vi "AI_InstantAI v2.vi"() -> ()   [LabVIEW 2013]
uses:
  <vilib>/Platform/TimedLoop/XDataNode/timing_clust.ctl
  <vilib>/Platform/TimedLoop/XDataNode/nitl_modes.ctl
  <vilib>/Platform/TimedLoop/XDataNode/wakeup.ctl
  <vilib>/platform/TimedLoop/XDataNode/XDataNode.xnode
  <vilib>/Platform/TimedLoop/XDataNode/XDNodeRunTimeDep.lvlib
panel:
  in  "Samples":i32
  out "loop time":dbl format="%.6g"
  in  "Tab Control":enum32{"Graph0", "Graph1", "Graph2"}(tab)
  out "Graph0":dbl[][](graph)
  out "Ch0":dbl[](array[numeric])
  out "Ch1":dbl[](array[numeric])
  out "Ch2":dbl[](array[numeric])
  out "Ch3":dbl[](array[numeric])
  out "Ch4":dbl[](array[numeric])
  out "Ch5":dbl[](array[numeric])
  out "Ch6":dbl[](array[numeric])
  out "Ch7":dbl[](array[numeric])
  out "error 0":errorcluster
  out "Ch7-1":dbl[](array[numeric])
  out "Ch6-1":dbl[](array[numeric])
  out "Ch5-1":dbl[](array[numeric])
  out "Ch4-1":dbl[](array[numeric])
  out "Ch3-1":dbl[](array[numeric])
  out "Ch2-1":dbl[](array[numeric])
  out "Ch1-1":dbl[](array[numeric])
  out "Ch0-1":dbl[](array[numeric])
  out "error 1":errorcluster
  out "Graph1":dbl[][](graph)
  out "loops":bool
  in  "stop":bool
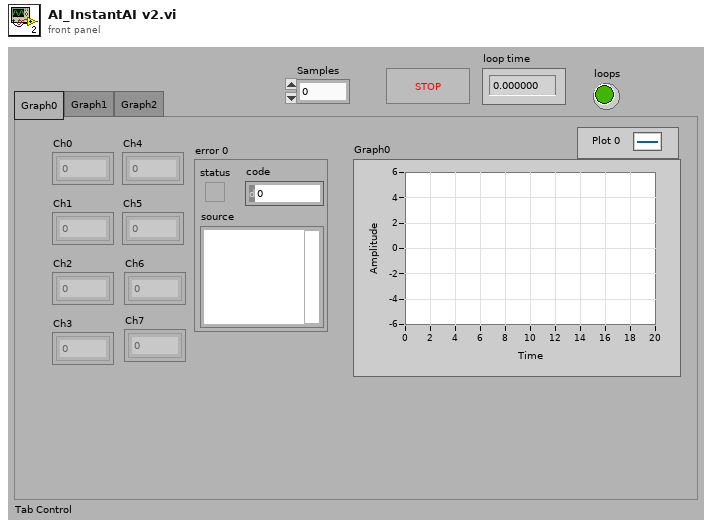
[diagram p1: front panel]
types:
  T1 = typedef "XDNodeRunTimeDep.lvlib/timing_clust.ctl" = cluster{"Expected End [f-1]":u64, "Actual End [f-1]":u64, "Finished Late? [f-1]":bool, "Expected End [i-1]":u64, "Actual End [i-1]":u64, "Finished Late? [i-1]":bool, "Expected Start [i]":u64, "Actual Start [i]":u64, "Expected Start [f]":u64, "Actual Start [f]":u64, "Source Name":string, "Structure Name":string, "Period":i64, "Deadline":i64, "Offset":i64, "Start":i64, "Priority":i32, "Timeout":i32, "Mode":T2, "Wakeup Reason":T3, "Error":errorcluster, "Source Type":string, "Secondary Source Type":string, "Global End Time":u64, "Global Start Time":u64, "Frame Duration":u64, "Iteration Duration":u64, "Assigned CPU":i32, "I/O Scan Engine Mode":u32}
  T2 = typedef "XDNodeRunTimeDep.lvlib/nitl_modes.ctl" = enum32{"No Change", "Process missed periods, maintain original phase", "Discard missed periods, maintain original phase", "Process missed periods, ignore original phase", "Discard missed periods, ignore original phase"}
  T3 = typedef "XDNodeRunTimeDep.lvlib/wakeup.ctl" = enum32{"Normal", "Aborted", "Asynchronous wakeup", "Timing source error", "Timed loop error", "Timeout"}
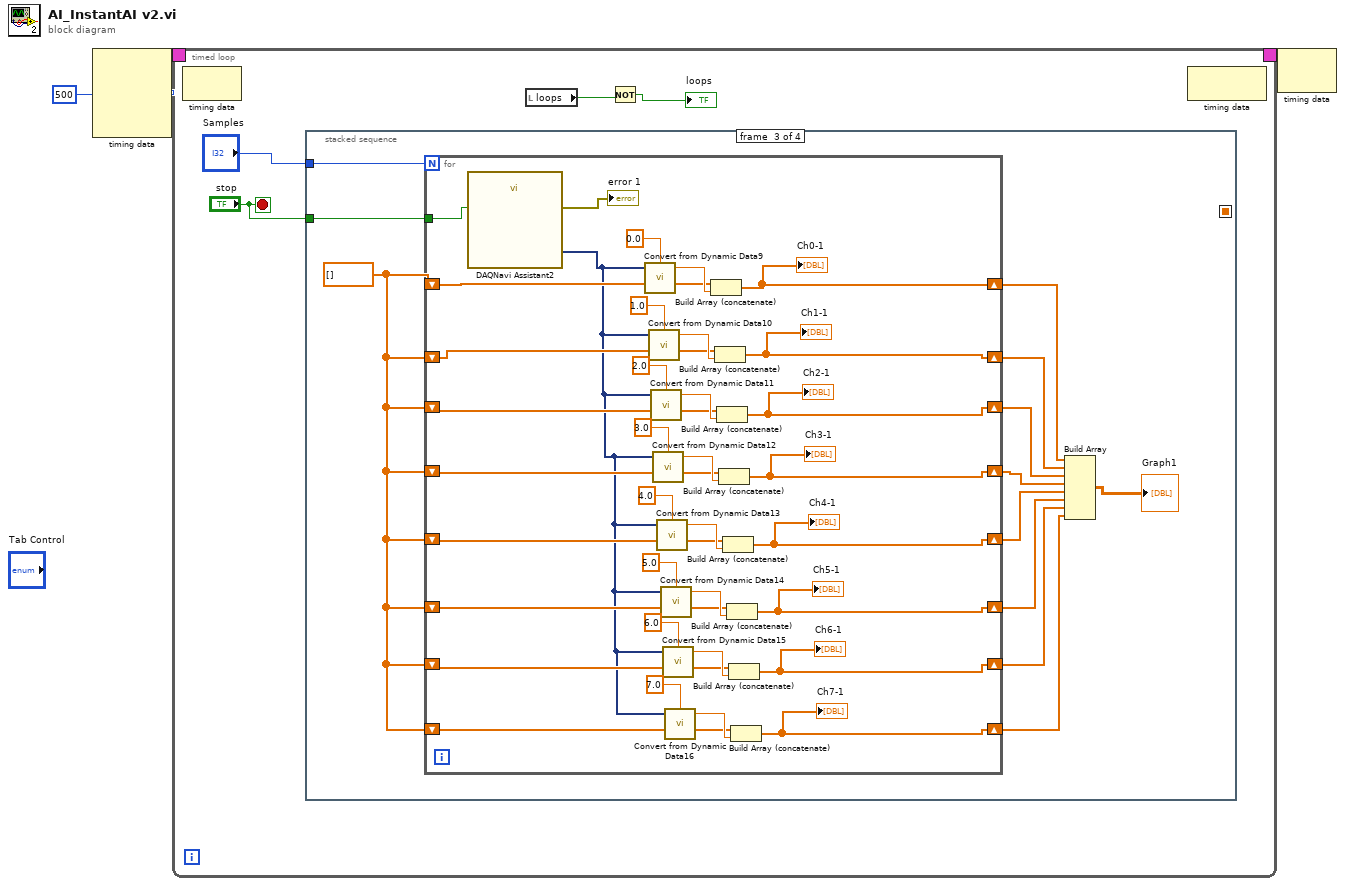
[diagram p0: block diagram]
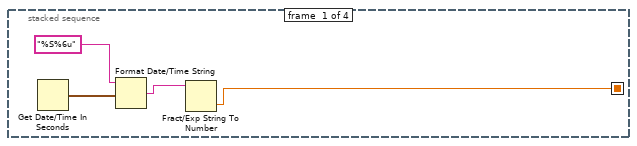
[diagram p2: hidden frame]
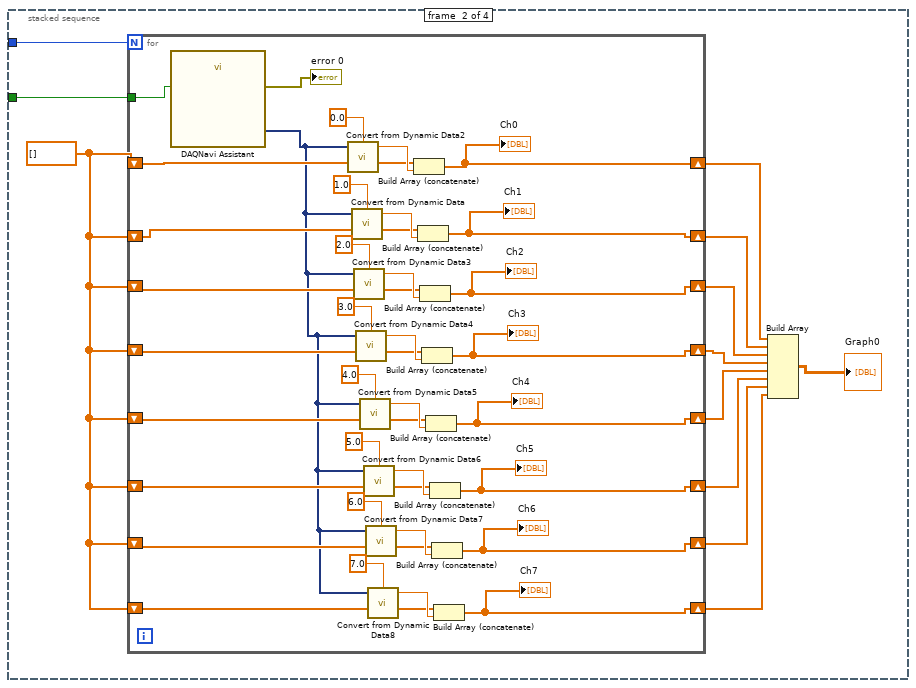
[diagram p3: hidden frame]
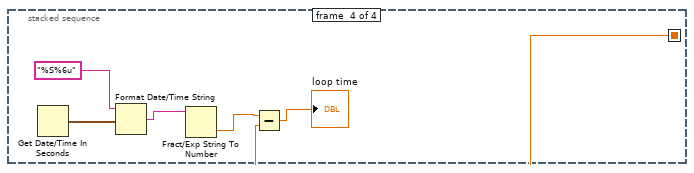
[diagram p4: hidden frame]
diagram:
  n1 = node-c288(500) -> (w3:T1)  [unwired: 3 in]
  n2 = timed-loop {
    timing: w3 -> [_]
    timing-out: [_] -> w2
    stop <- "stop" stop-if-true
    n3 = node-c288() -> ()  [unwired: 1 in, 1 out]
    n4 = stacked-sequence {
      seq-local: [w8 _ _ _] -> [_ _ _ w106]
      tunnel: "stop" -> [_ w23 w70 _]
      tunnel: "Samples" -> [_ w12 w59 _]
      frame #0 {
        n5 = Get Date/Time In Seconds() -> (seconds since 1Jan1904=w10:timestamp)
        n6 = Format Date/Time String(time format string (%c)="%S%6u", seconds (now)=w10) -> (date/time string=w9:string)  [unwired: 1 in]
        n7 = Fract/Exp String To Number(string=w9) -> (number=w8:dbl)  [unwired: 3 in, 1 out]
      }
      frame #1 {
        w22 = dbl[] []
        n8 = for {
          N: w12 -> [_]
          tunnel: w23 -> [w24]
          shift-right: [w54] -> w21
          shift-left: w22 -> [w55]
          shift-right: [w51] -> w20
          shift-left: w22 -> [w50]
          shift-right: [w47] -> w19
          shift-left: w22 -> [w46]
          shift-right: [w43] -> w15
          shift-left: w22 -> [w42]
          shift-right: [w32] -> w14
          shift-left: w22 -> [w33]
          shift-right: [w31] -> w16
          shift-left: w22 -> [w28]
          shift-right: [w30] -> w17
          shift-left: w22 -> [w27]
          shift-right: [w29] -> w18
          shift-left: w22 -> [w26]
          n9 = call "DAQNavi Assistant"("stop(true)"=w24) -> ("error out"=→"error 0":errorcluster, "data out(DDT)"=w25:dynamicdata)  [unwired: 1 in, 16 out]
          n10 = call "Convert from Dynamic Data2"("Dynamic Data Type"=w25, "Channel"=0.0) -> ("Scalar"=w56:dbl)  [unwired: 2 in]
          n11 = call "Convert from Dynamic Data"("Dynamic Data Type"=w25, "Channel"=1.0) -> ("Scalar"=w52:dbl)  [unwired: 2 in]
          n12 = call "Convert from Dynamic Data3"("Dynamic Data Type"=w25, "Channel"=2.0) -> ("Scalar"=w48:dbl)  [unwired: 2 in]
          n13 = call "Convert from Dynamic Data4"("Dynamic Data Type"=w25, "Channel"=3.0) -> ("Scalar"=w44:dbl)  [unwired: 2 in]
          n14 = call "Convert from Dynamic Data5"("Dynamic Data Type"=w25, "Channel"=4.0) -> ("Scalar"=w40:dbl)  [unwired: 2 in]
          n15 = call "Convert from Dynamic Data6"("Dynamic Data Type"=w25, "Channel"=5.0) -> ("Scalar"=w38:dbl)  [unwired: 2 in]
          n16 = call "Convert from Dynamic Data7"("Dynamic Data Type"=w25, "Channel"=6.0) -> ("Scalar"=w36:dbl)  [unwired: 2 in]
          n17 = call "Convert from Dynamic Data8"("Dynamic Data Type"=w25, "Channel"=7.0) -> ("Scalar"=w34:dbl)  [unwired: 2 in]
          n18 = Build Array (concatenate)(w55, w56) -> (w54:dbl[])
          "Ch0" <- w54
          n19 = Build Array (concatenate)(w50, w52) -> (w51:dbl[])
          "Ch1" <- w51
          n20 = Build Array (concatenate)(w46, w48) -> (w47:dbl[])
          "Ch2" <- w47
          n21 = Build Array (concatenate)(w42, w44) -> (w43:dbl[])
          "Ch3" <- w43
          n22 = Build Array (concatenate)(w33, w40) -> (w32:dbl[])
          "Ch4" <- w32
          n23 = Build Array (concatenate)(w28, w38) -> (w31:dbl[])
          "Ch5" <- w31
          n24 = Build Array (concatenate)(w27, w36) -> (w30:dbl[])
          "Ch6" <- w30
          n25 = Build Array (concatenate)(w26, w34) -> (w29:dbl[])
          "Ch7" <- w29
        }
        n26 = Build Array(w21, w20, w19, w15, w14, w16, w17, w18) -> (→"Graph0":dbl[][])
      }
      frame #2 {
        w69 = dbl[] []
        n27 = for {
          N: w59 -> [_]
          tunnel: w70 -> [w71]
          shift-right: [w101] -> w68
          shift-left: w69 -> [w102]
          shift-right: [w98] -> w67
          shift-left: w69 -> [w97]
          shift-right: [w94] -> w66
          shift-left: w69 -> [w93]
          shift-right: [w90] -> w62
          shift-left: w69 -> [w89]
          shift-right: [w79] -> w61
          shift-left: w69 -> [w80]
          shift-right: [w78] -> w63
          shift-left: w69 -> [w75]
          shift-right: [w77] -> w64
          shift-left: w69 -> [w74]
          shift-right: [w76] -> w65
          shift-left: w69 -> [w73]
          n28 = call "DAQNavi Assistant2"("stop(true)"=w71) -> ("error out"=→"error 1":errorcluster, "data out(DDT)"=w72:dynamicdata)  [unwired: 1 in, 16 out]
          n29 = call "Convert from Dynamic Data9"("Dynamic Data Type"=w72, "Channel"=0.0) -> ("Scalar"=w103:dbl)  [unwired: 2 in]
          n30 = call "Convert from Dynamic Data10"("Dynamic Data Type"=w72, "Channel"=1.0) -> ("Scalar"=w99:dbl)  [unwired: 2 in]
          n31 = call "Convert from Dynamic Data11"("Dynamic Data Type"=w72, "Channel"=2.0) -> ("Scalar"=w95:dbl)  [unwired: 2 in]
          n32 = call "Convert from Dynamic Data12"("Dynamic Data Type"=w72, "Channel"=3.0) -> ("Scalar"=w91:dbl)  [unwired: 2 in]
          n33 = call "Convert from Dynamic Data13"("Dynamic Data Type"=w72, "Channel"=4.0) -> ("Scalar"=w87:dbl)  [unwired: 2 in]
          n34 = call "Convert from Dynamic Data14"("Dynamic Data Type"=w72, "Channel"=5.0) -> ("Scalar"=w85:dbl)  [unwired: 2 in]
          n35 = call "Convert from Dynamic Data15"("Dynamic Data Type"=w72, "Channel"=6.0) -> ("Scalar"=w83:dbl)  [unwired: 2 in]
          n36 = call "Convert from Dynamic Data16"("Dynamic Data Type"=w72, "Channel"=7.0) -> ("Scalar"=w81:dbl)  [unwired: 2 in]
          n37 = Build Array (concatenate)(w102, w103) -> (w101:dbl[])
          "Ch0-1" <- w101
          n38 = Build Array (concatenate)(w97, w99) -> (w98:dbl[])
          "Ch1-1" <- w98
          n39 = Build Array (concatenate)(w93, w95) -> (w94:dbl[])
          "Ch2-1" <- w94
          n40 = Build Array (concatenate)(w89, w91) -> (w90:dbl[])
          "Ch3-1" <- w90
          n41 = Build Array (concatenate)(w80, w87) -> (w79:dbl[])
          "Ch4-1" <- w79
          n42 = Build Array (concatenate)(w75, w85) -> (w78:dbl[])
          "Ch5-1" <- w78
          n43 = Build Array (concatenate)(w74, w83) -> (w77:dbl[])
          "Ch6-1" <- w77
          n44 = Build Array (concatenate)(w73, w81) -> (w76:dbl[])
          "Ch7-1" <- w76
        }
        n45 = Build Array(w68, w67, w66, w62, w61, w63, w64, w65) -> (→"Graph1":dbl[][])
      }
      frame #3 {
        n46 = Get Date/Time In Seconds() -> (seconds since 1Jan1904=w108:timestamp)
        n47 = Format Date/Time String(time format string (%c)="%S%6u", seconds (now)=w108) -> (date/time string=w109:string)  [unwired: 1 in]
        n48 = Fract/Exp String To Number(string=w109) -> (number=w110:dbl)  [unwired: 3 in, 1 out]
        n49 = Subtract(x=w110, y=w106) -> (x-y=→"loop time":dbl)
      }
    }
    n50 = local read "loops"() -> (w7:bool)
    n51 = Not(x=w7) -> (.not. x?=→"loops":bool)
    n52 = node-c288() -> ()  [unwired: 1 in, 1 out]
  }
  n53 = node-c288(w2) -> ()  [unwired: 1 out]
